vi "RemoveKnown.vi"(6 "Status":refnum<vi>, 8 "error in (no error)":errorcluster, 10 "filenames":string[](array[string]), 11 "Working Dir":path) -> (0 "error out":errorcluster, 1 "Known Found?":bool, 2 "Filenames Out":string[](array[string]), 3 "Working Dir Out":path, 4 "Tags Removed":string[](array[string]))   [LabVIEW 2022 SP3]
uses:
  TypeDefs/Tag Cmd.ctl
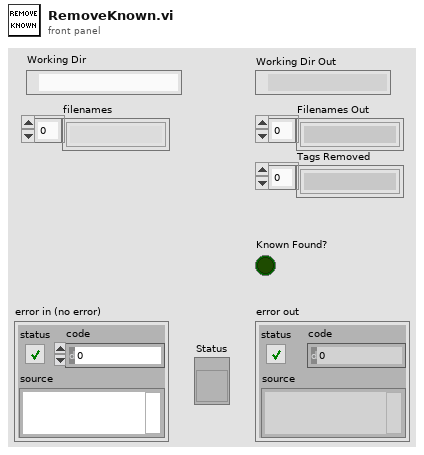
[diagram p1: front panel]
types:
  T1 = typedef "Tag Cmd.ctl" = enum16{"Init", "Get Known", "Set Known"}
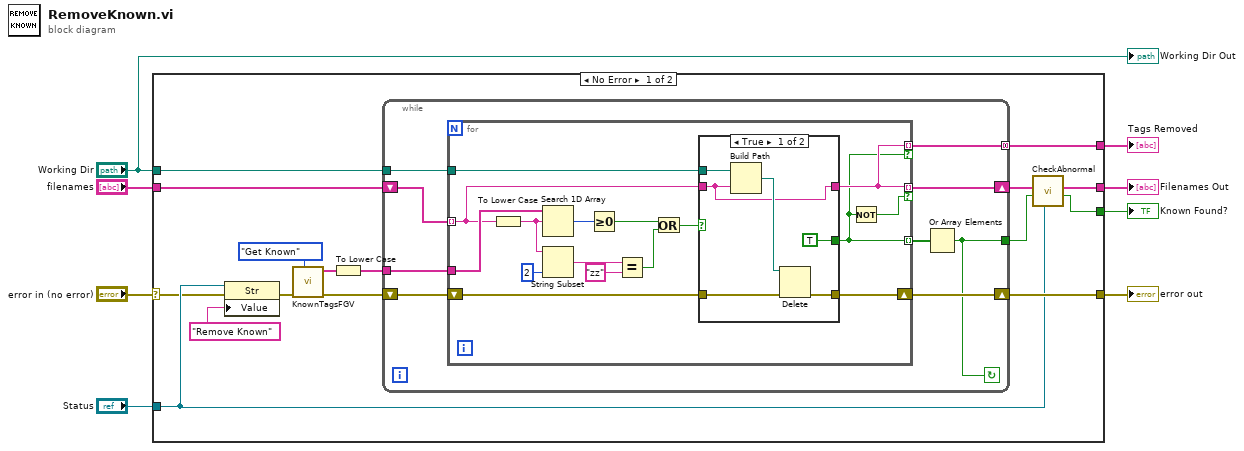
[diagram p0: block diagram]
diagram:
  n1 = case shown="No Error" "error in (no error)" {
    selector: "error in (no error)" -> [w9 w58]
    tunnel: "filenames" -> [w22 _]
    tunnel: [w20 w58] -> w7
    tunnel: "Working Dir" -> [w19 _]
    tunnel: [w15 _] -> w5
    tunnel: [w13 _] -> w4
    tunnel: "Status" -> [w12 _]
    tunnel: [w10 _] -> w2
    frame No Error {
      n2 = property class="Str"(reference=w12, error in=w9, "Value"="Remove Known") -> (error out=w18:errorcluster)  [unwired: 1 out]
      n3 = call "KnownTagsFGV.vi"("Tag Cmd"=Tag_Cmd."Get Known", "error in (no error)"=w18) -> ("error out"=w23:errorcluster, "Known Tags"=w21:string[])  [unwired: 8 in]
      n4 = To Lower Case(string=w21) -> (all lower case string=w11:string[])
      n5 = while {
        tunnel: w11 -> [w31]
        tunnel: w19 -> [w29]
        tunnel: [w26] -> w14
        shift-right: [w30] -> w20
        shift-left: w23 -> [w33]
        shift-right: [w27] -> w16
        shift-left: w22 -> [w32]
        tunnel: [w25] -> w10 mode=concatenating
        stop <- w26 continue-if-true
        n6 = for {
          shift-right: [w47] -> w30
          shift-left: w33 -> [w48]
          tunnel: w32 -> [w45] mode=indexing
          tunnel: w31 -> [w49]
          tunnel: w29 -> [w46]
          tunnel: [w42] -> w28 mode=indexing
          tunnel: [w43] -> w27 mode=indexing if=w44
          tunnel: [w43] -> w25 mode=indexing if=w42
          n7 = To Lower Case(string=w45) -> (all lower case string=w40:string)
          n8 = Search 1D Array(1D array=w49, element=w40) -> (index of element=w41:i32)  [unwired: 1 in]
          n9 = String Subset(string=w40, length (rest)=2 ("length (rest)")) -> (substring=w38:string)  [unwired: 1 in]
          n10 = Greater Or Equal To 0?(x=w41) -> (x >= 0?=w35:bool)
          n11 = Equal?(x=w38, y="zz") -> (x = y?=w34:bool)
          n12 = Or(x=w35, y=w34) -> (x .or. y?=w36:bool)
          n13 = case shown="True" w36 {
            tunnel: w48 -> [w55 w57]
            tunnel: [w54 w57] -> w47
            tunnel: w46 -> [w53 _]
            tunnel: w45 -> [w50 w56]
            tunnel: [TRUE _] -> w42
            tunnel: [w50 w56] -> w43
            frame True {
              n14 = Build Path(base path=w53, name or relative path=w50) -> (appended path=w52:path)
              n15 = Delete(path (use dialog)=w52, error in=w55) -> (error out=w54:errorcluster)  [unwired: 3 in, 2 out]
            }
            frame False {
            }
          }
          n16 = Not(x=w42) -> (.not. x?=w44:bool)
        }
        n17 = Or Array Elements(Boolean array=w28) -> (logical OR=w26:bool)
      }
      n18 = call "CheckAbnormal.vi"("Status"=w12, "Known Found?"=w14, "Filenames"=w16) -> ("Ignore"=w13:bool, "Filenames out"=w15:string[])  [unwired: 7 in]
    }
    frame Error {
    }
  }
  "error out" <- w7
  "Known Found?" <- w4
  "Filenames Out" <- w5
  "Tags Removed" <- w2
  "Working Dir Out" <- "Working Dir"
